vi "RemoveItemsBelongingToLibrary.vi"(7 "FileDependency In":map{path, T1}(c390), 9 "EvenSubLibraries":bool, 11 "LibraryDependency In":map{path, T3}(c390)) -> (3 "LibraryDependency Out":map{path, T3}(c390))   [LabVIEW 2020, in "DependencyViewer.lvlib"]
uses:
  DependencyViewer.lvlib
  LibraryDependentInfo.vi
  <vilib>/Utility/lvfile.llb/FT_FileTypes.ctl
  FileDependencyType.ctl
  <vilib>/Utility/lvfile.llb/NI_FileType.lvlib
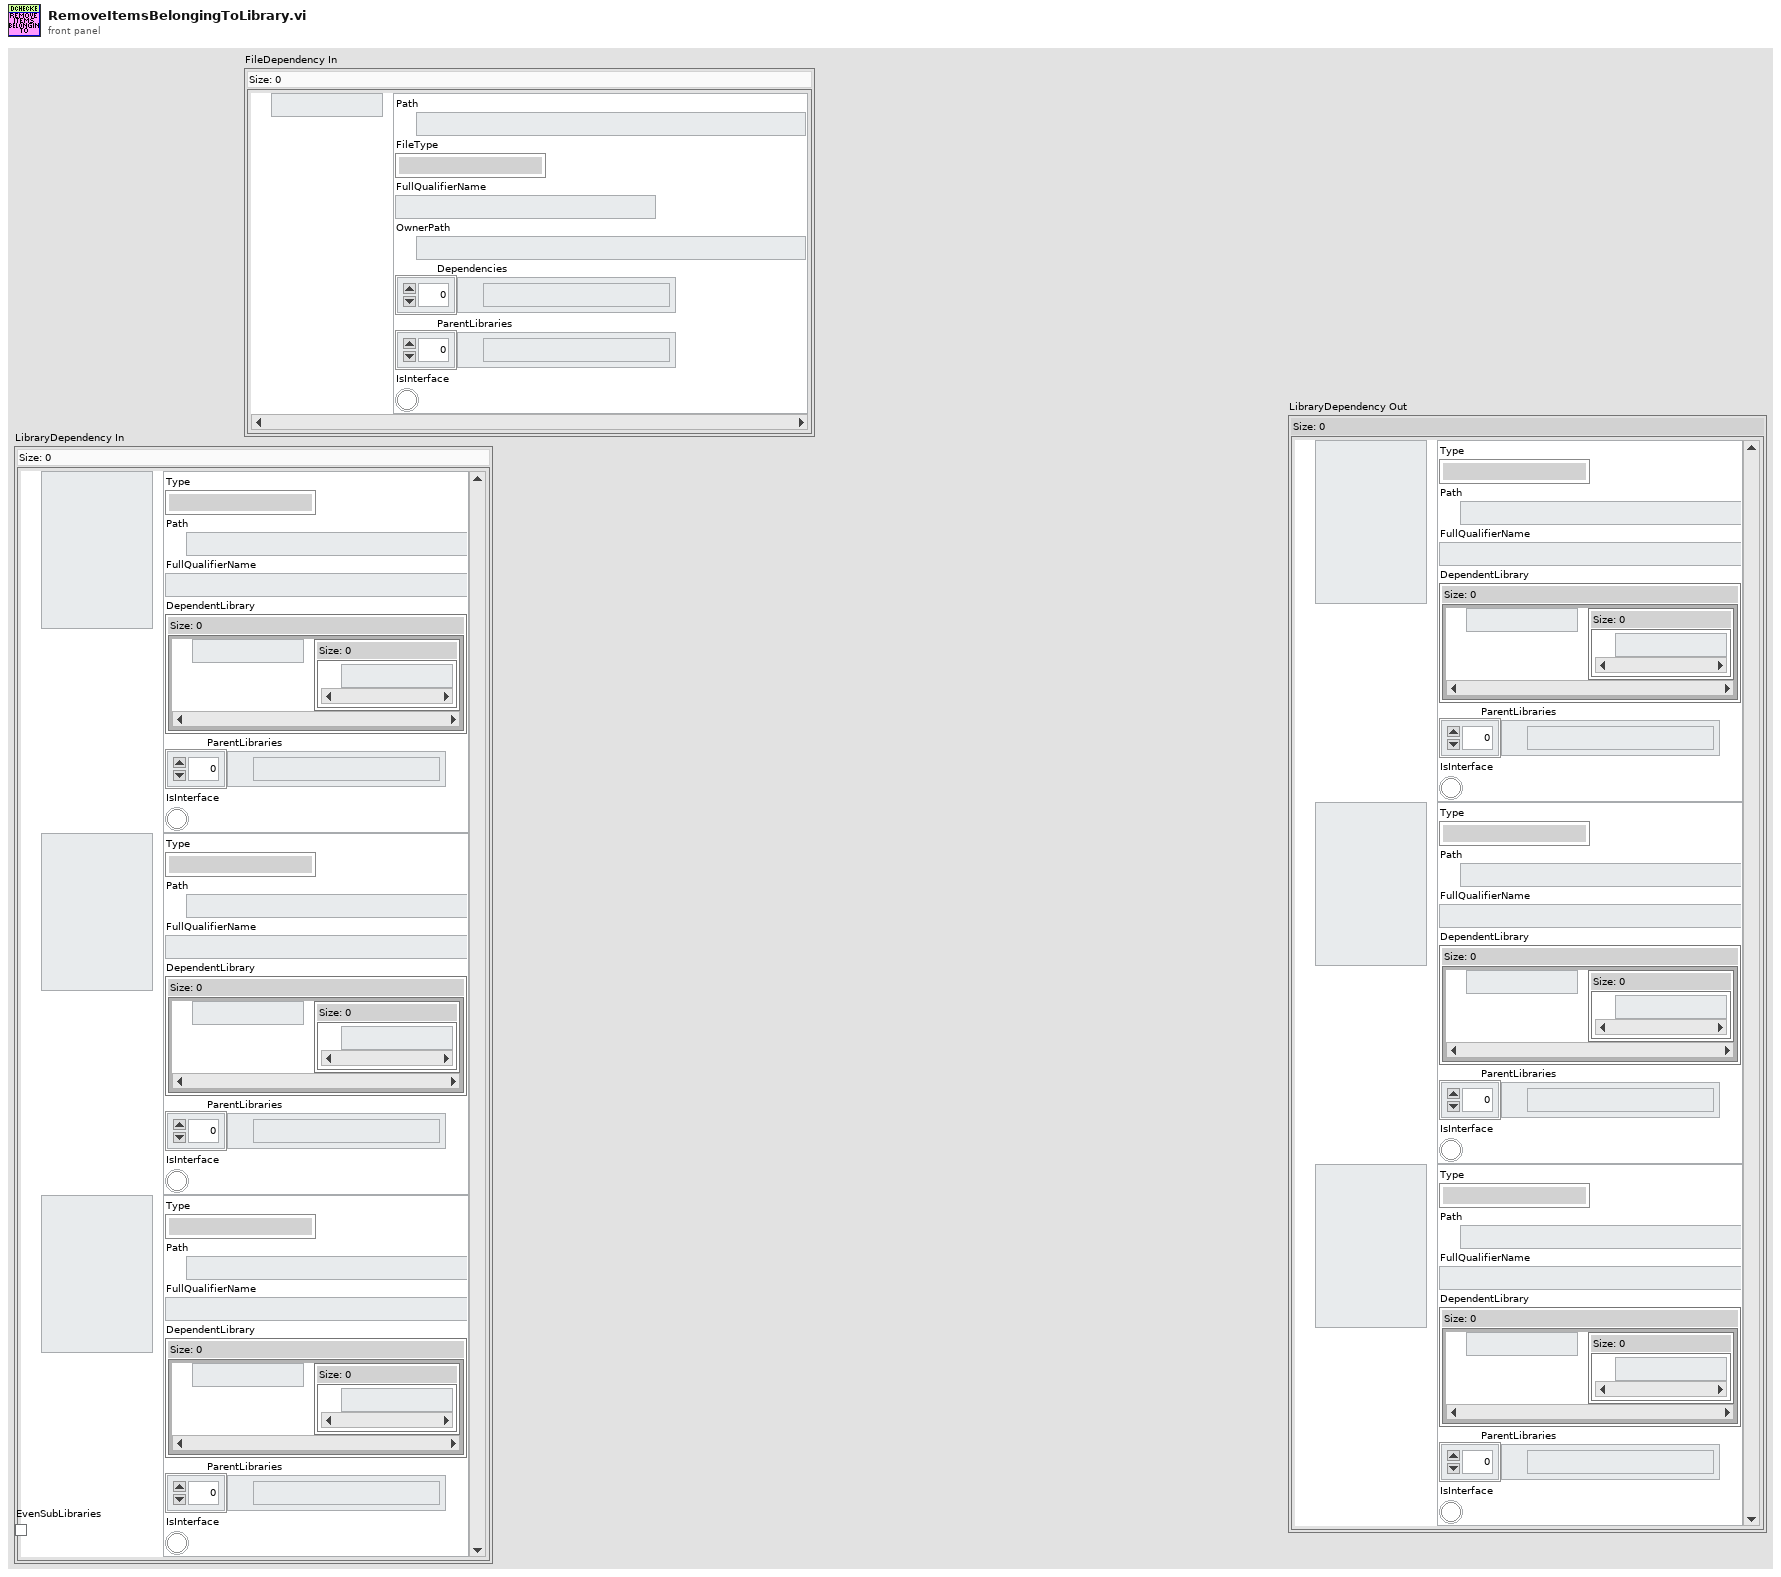
[diagram p1: front panel]
types:
  T1 = typedef "DependencyViewer.lvlib/FileDependencyType.ctl" = cluster{"Path":path, "FileType":T2, "FullQualifierName":string, "OwnerPath":path, "Dependencies":path[], "ParentLibraries":path[], "IsInterface":bool}
  T2 = typedef "NI_FileType.lvlib/FT_FileTypes.ctl" = enum32{"Invalid file/path", "Unknown type", "Instrument", "Control", "Polymorphic VI", "Project", "Library", "LVClass", "XControl", "XNode", "CIN", "Run-time menu", "Palette menu", "LLB", "Shortcut", "Directory", "Class Private Data Control", "Statechart", "MathScript .m file", "Ladder Diagram", "LVLibp"}
  T3 = typedef "DependencyViewer.lvlib/LibraryDependentInfo.vi" = cluster{"Type":T2, "Path":path, "FullQualifierName":string, "DependentLibrary":map{path, set{path}}, "ParentLibraries":path[], "IsInterface":bool}
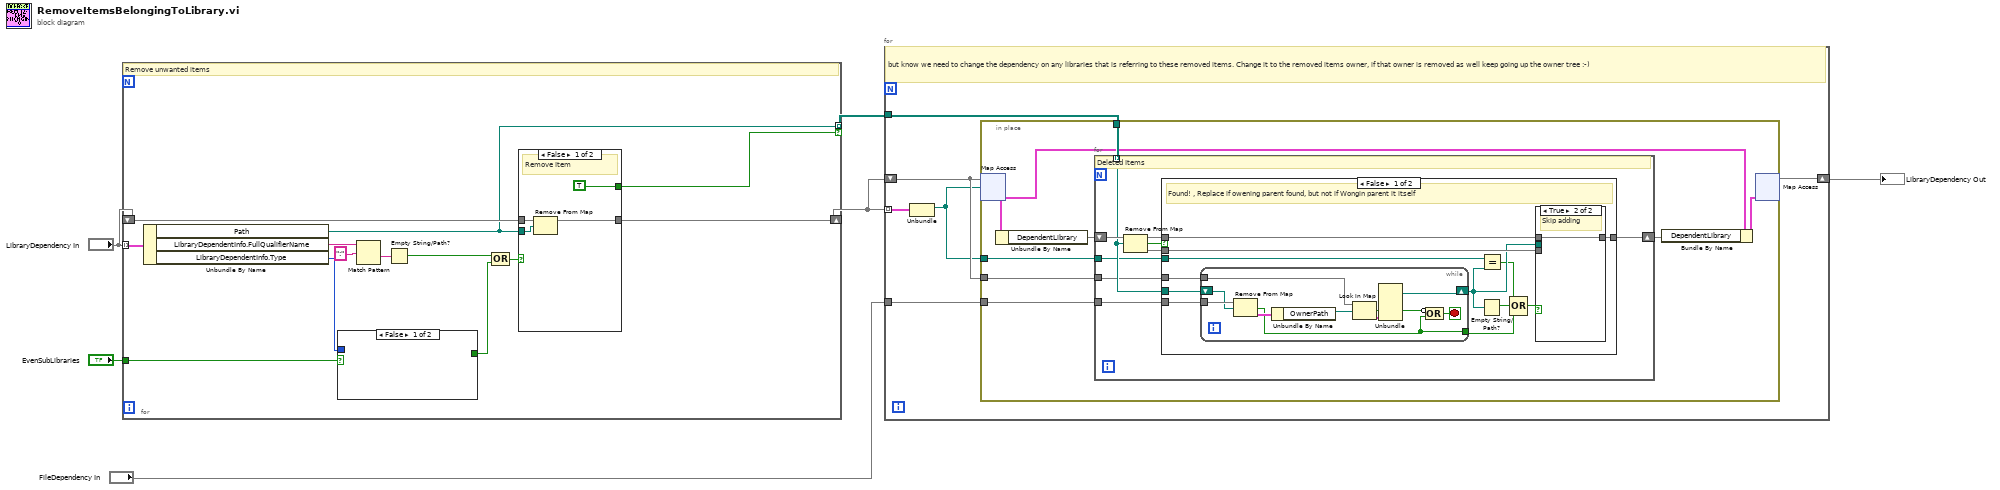
[diagram p0: block diagram]
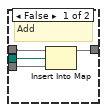
[diagram p2: hidden frame]
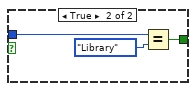
[diagram p4: hidden frame]
diagram:
  n1 = for {
    tunnel: "LibraryDependency In" -> [w19] mode=indexing
    shift-right: [w16] -> w4
    shift-left: "LibraryDependency In" -> [w17]
    tunnel: "EvenSubLibraries" -> [w11]
    tunnel: [w8] -> w3 mode=indexing if=w7
    # "Remove unwanted items"
    n2 = Unbundle By Name(w19) -> ("Path"=w8:path, "LibraryDependentInfo.FullQualifierName"=w15:string, "LibraryDependentInfo.Type"=w18:T2)
    n3 = case shown="False" w11 {
      tunnel: w18 -> [_ w22]
      tunnel: [_ w20] -> w10
      frame False {
      }
      frame True {
        n4 = Equal?(x=w22, y=FT_FileTypes."Library") -> (x = y?=w20:bool)
      }
    }
    n5 = Match Pattern(string=w15, regular expression=":") -> (after substring=w13:string)  [unwired: 1 in, 3 out]
    n6 = Empty String/Path?(string/path=w13) -> (empty?=w12:bool)
    n7 = Compound Arithmetic op=OR(w12, w10) -> (w9:bool)
    n8 = case shown="False" w9 {
      tunnel: w17 -> [w26 w27]
      tunnel: w8 -> [w25 _]
      tunnel: [w24 w27] -> w16
      tunnel: [TRUE _] -> w7
      frame False {
        # "Remove Item"
        n9 = Remove From Map(10:w25, 11:w26) -> (3:w24:map{path, T3})  [unwired: 2 out]
      }
      frame True {
        # "Keep this item"
      }
    }
  }
  n10 = for {
    tunnel: w4 -> [w33] mode=indexing
    shift-right: [w29] -> w1
    shift-left: w4 -> [w30]
    tunnel: w3 -> [w32]
    tunnel: "FileDependency In" -> [w31]
    # "but know we need to change the dependency on any libraries that is referring to these removed items. Change it to the removed items owner, if that owner is removed as well keep going up the owner tree :-)"
    n11 = Unbundle(w33) -> ("Path"=w28:path)  [unwired: 1 out]
    n12 = in-place {
      in-place-border: w32 -> [w40]
      in-place-border: w31 -> [w36]
      in-place-border: w30 -> [w35]
      in-place-border: w28 -> [w34]
      n13 = in-place-map #1(w30, w28) -> (w39:T3)  [unwired: 1 in, 1 out]
      n14 = Unbundle By Name(w39) -> ("DependentLibrary"=w41:map{path, set{path}})
      n15 = for {
        shift-right: [w48] -> w38
        shift-left: w41 -> [w50]
        tunnel: w40 -> [w45] mode=indexing
        tunnel: w36 -> [w46]
        tunnel: w35 -> [w43]
        tunnel: w34 -> [w42]
        # "Deleted Items"
        n16 = Remove From Map(10:w45, 11:w50) -> (1:w44:set{path}, 2:w49:bool, 3:w47:map{path, set{path}})
        n17 = case shown="False" w49 {
          tunnel: [w59 w78] -> w48
          tunnel: w47 -> [w60 w78]
          tunnel: w46 -> [w62 _]
          tunnel: w45 -> [w61 _]
          tunnel: w44 -> [w58 _]
          tunnel: w43 -> [w57 _]
          tunnel: w42 -> [w52 _]
          frame False {
            # "Found! , Replace if owening parent found, but not if Wongin parent it itself"
            n18 = while {
              shift-right: [w69] -> w53
              shift-left: w61 -> [w76]
              tunnel: w62 -> [w77]
              tunnel: w57 -> [w73]
              tunnel: [w68] -> w55
              stop <- w71 stop-if-true
              n19 = Remove From Map(10:w76, 11:w77) -> (1:w75:T1, 2:w68:bool)  [unwired: 1 out]
              n20 = Unbundle By Name(w75) -> ("OwnerPath"=w74:path)
              n21 = Look In Map(map=w73, key=w74) -> (key not found?=w72:bool, value=w70:T3)  [unwired: 1 in]
              n22 = Unbundle(w70) -> ("Path"=w69:path)  [unwired: 5 out]
              n23 = Compound Arithmetic op=OR(invert w72, w68) -> (w71:bool)
            }
            n24 = Empty String/Path?(string/path=w53) -> (empty?=w56:bool)
            n25 = Equal?(x=w52, y=w53) -> (x = y?=w51:bool)
            n26 = Compound Arithmetic op=OR(w51, w56, w55) -> (w54:bool)
            n27 = case shown="True" w54 {
              tunnel: w60 -> [w66 w67]
              tunnel: [w65 w67] -> w59
              tunnel: w58 -> [w64 _]
              tunnel: w53 -> [w63 _]
              frame False {
                # "Add"
                n28 = Insert Into Map(map in=w66, key=w63, value=w64) -> (map out=w65:map{path, set{path}})  [unwired: 2 out]
              }
              frame True {
                # "Skip adding"
              }
            }
          }
          frame True {
            # "Not found"
          }
        }
      }
      n29 = Bundle By Name(cluster=w39, "DependentLibrary"=w38) -> (w37:T3)
      n30 = in-place-map #1(w37) -> (w29:map{path, T3})  [unwired: 1 in, 2 out]
    }
  }
  "LibraryDependency Out" <- w1
